vi "PushPullMachine_sub.vi"(0 "Notify?":bool) -> (1 "notification":string="53 got Queue", 2 "Shift#":dbl)   [LabVIEW 2024]
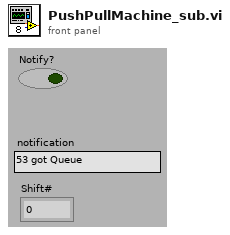
[diagram p1: front panel]
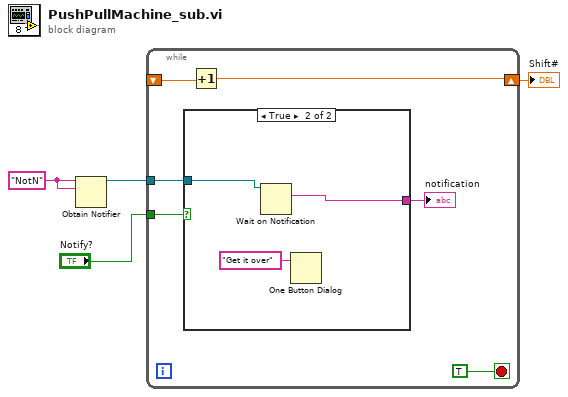
[diagram p0: block diagram]
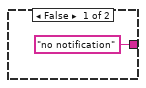
[diagram p2: hidden frame]
diagram:
  w4 = "NotN" ("name (unnamed)")
  n1 = Obtain Notifier(name (unnamed)=w4, notification data type=w4) -> (notifier out=w3:refnum<notifier>)  [unwired: 2 in, 2 out]
  n2 = while {
    tunnel: w3 -> [w9]
    tunnel: "Notify?" -> [w8]
    shift-right: [w5] -> w1
    shift-left: _ -> [w6]
    stop <- TRUE stop-if-true
    n3 = case shown="True" w8 {
      tunnel: ["no notification" ("name (unnamed)") w14] -> w10
      tunnel: w9 -> [_ w13]
      frame False {
      }
      frame True {
        n4 = Wait on Notification(notifier=w13) -> (notification=w14:string)  [unwired: 3 in, 3 out]
        n5 = One Button Dialog(message="Get it over") -> ()  [unwired: 1 in, 1 out]
      }
    }
    "notification" <- w10
    n6 = Increment(x=w6) -> (x+1=w5:dbl)
  }
  "Shift#" <- w1
